vi "ExDataFileToSpreadsheet.vi"() -> ()   [LabVIEW 2010]
uses:
  <vilib>/Utility/file.llb/Write To Spreadsheet File (DBL).vi
panel:
  in  "Input File Name":path
  in  "Spreadsheet File Name (include .xls extension)":path
  in  "Input File Operation":u32=6
  in  "Input FileType":u32=67371008
  out "error out":errorcluster
  in  "error in (no error)":errorcluster
  # "ExDataFileToSpreadsheet.vi\nThis VI will open the input file and save it to the\noutput file.  Note that the full path names\nmust be provided for both input and output files."
  # "TIF   = 67174400\n  SPE = 67371008\n  PMI  = 67436544"
  # "6 = Read Only"
  # "NOTICE\n\nTHIS VI REQUIRES THAT THE TOOLKIT\nBE UNLOADED BY RUNNING THE\n VI EXCLOSEGLOBALCAM.VI\n BEFORE LEAVING LABVIEW."
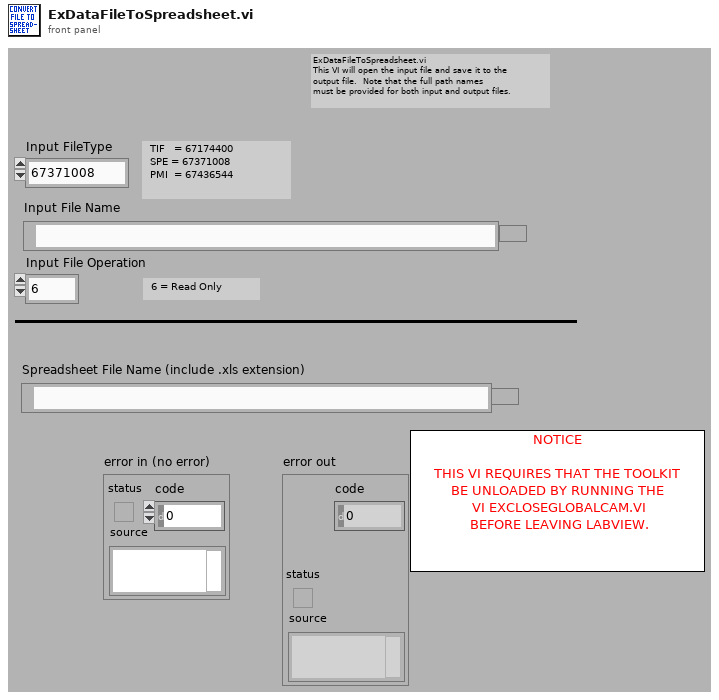
[diagram p1: front panel]
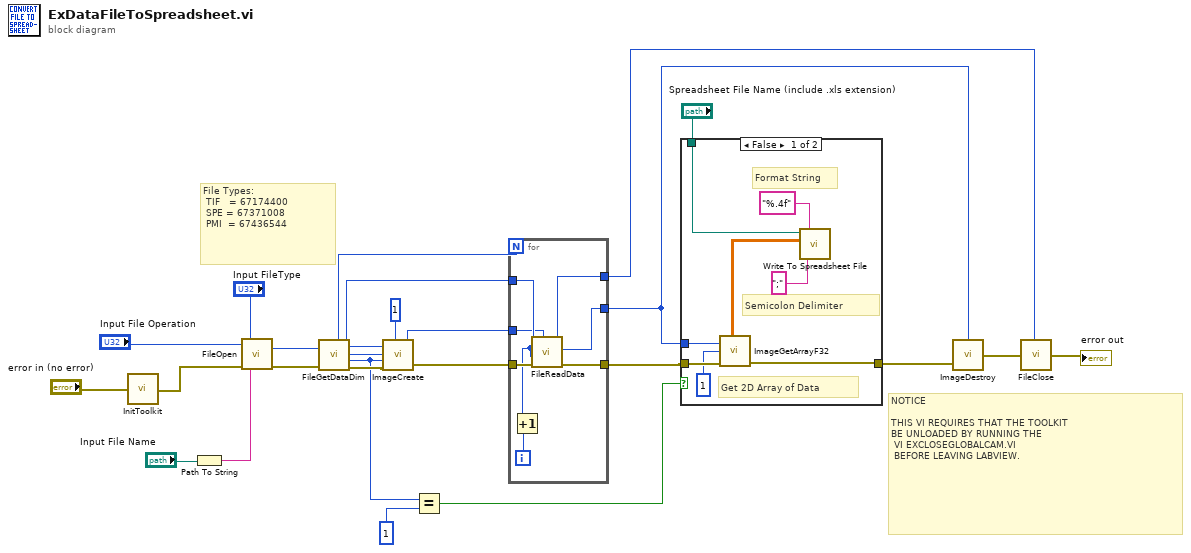
[diagram p0: block diagram]
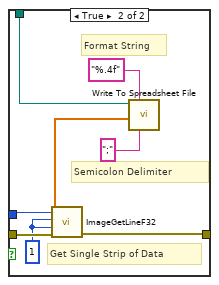
[diagram p2: hidden frame]
diagram:
  # "NOTICE\n\nTHIS VI REQUIRES THAT THE TOOLKIT\nBE UNLOADED BY RUNNING THE\n VI EXCLOSEGLOBALCAM.VI\n BEFORE LEAVING LABVIEW."
  # "File Types:\n TIF   = 67174400\n SPE = 67371008\n PMI  = 67436544"
  n1 = call <userlib>:"InitToolkit.vi"("error in"="error in (no error)") -> ("error out"=w14:errorcluster)
  n2 = Path To String(path="Input File Name") -> (string=w5:string)
  n3 = call <userlib>:"FileOpen.vi"("error in"=w14, "File Operations"="Input File Operation", "FileName"=w5, "File Type"="Input FileType") -> ("error out"=w24:errorcluster, "File Handle"=w23:u32)
  n4 = call <userlib>:"FileGetDataDim.vi"("File Handle"=w23, "error in"=w24) -> ("Number of Frames"=w21:u32, "Data Type"=w7:u32, "File Handle"=w19:u32, "X dim"=w9:u32, "Y dim"=w6:u32, "error out"=w22:errorcluster)
  n5 = call <userlib>:"ImageCreate.vi"("X dimension"=w9, "Y dimension"=w6, "Data Type"=w7, "error in"=w22, "Number Of Frames"=1) -> ("Image Handle"=w18:u32, "error out"=w4:errorcluster)
  n6 = Equal?(x=w7, y=1) -> (x = y?=w12:bool)
  n7 = for {
    N: w21 -> [_]
    tunnel: w4 -> [w34]
    tunnel: w19 -> [w33]
    tunnel: w18 -> [w32]
    tunnel: [w27] -> w3
    tunnel: [w29] -> w17
    tunnel: [w28] -> w8
    i -> [w31]
    n8 = Increment(x=w31) -> (x+1=w30:i32)
    n9 = call <userlib>:"FileReadData.vi"("File Handle"=w33, "Start Frame"=w30, "End Frame"=w30, "error in"=w34, "Image Handle"=w32) -> ("File Handle"=w29:u32, "Image Handle"=w28:u32, "error out"=w27:errorcluster)
  }
  n10 = case shown="False" w12 {
    tunnel: w3 -> [w39 w49]
    tunnel: [w36 w50] -> w2
    tunnel: w8 -> [w35 w48]
    tunnel: "Spreadsheet File Name (include .xls extension)" -> [w40 w43]
    frame False {
      # "Semicolon Delimiter"
      # "Format String"
      # "Get 2D Array of Data"
      n11 = call <userlib>:"ImageGetArrayF32.vi"("error in"=w39, "Z position"=1, "Image Handle"=w35) -> ("error out"=w36:errorcluster, "Array Float 32"=w37:sgl[][])  [unwired: 1 out]
      n12 = call-poly <vilib>:"Write To Spreadsheet File.vi"("delimiter (\\t)"=";", "format (%.3f)"="%.4f", "2D data"=w37, "file path (dialog if empty)"=w40) -> ()  [unwired: 4 in, 1 out]
    }
    frame True {
      w47 = 1
      # "Semicolon Delimiter"
      # "Format String"
      # "Get Single Strip of Data"
      n13 = call <userlib>:"ImageGetLineF32.vi"("error in"=w49, "Z Position"=w47, "Y Position"=w47, "Data Handle"=w48) -> ("error out"=w50:errorcluster, "Array F32"=w44:sgl[])  [unwired: 1 out]
      n14 = call-poly <vilib>:"Write To Spreadsheet File.vi"("delimiter (\\t)"=";", "format (%.3f)"="%.4f", "1D data"=w44, "file path (dialog if empty)"=w43) -> ()  [unwired: 4 in, 1 out]
    }
  }
  n15 = call <userlib>:"ImageDestroy.vi"("error in"=w2, "Data handle"=w8) -> ("error out"=w16:errorcluster)
  n16 = call <userlib>:"FileClose.vi"("error in"=w16, "File Handle"=w17) -> ("error out"=→"error out":errorcluster)
